vi "AR Drone Controller.vi"() -> ()   [LabVIEW 2014]
doc: "Very simple example showing how to use the base VIs to control the AR Drone and receive and display navigation data."
uses:
  <vilib>/LVH/AR Drone Toolkit/Decode NavData/Typedefs/NavData Demo.ctl
  Control 1.ctl
  <vilib>/LVH/AR Drone Toolkit/AR Drone.lvlib
panel:
  out "Video Stream":picture
  out "Battery Remaining":T1 scale=0.0..100.0
  out "NavData Out":T2
  in  "Control Cluster":T3 {"Yaw Speed" scale=-1.0..1.0; "Vertical Speed" scale=-1.0..1.0; "Pitch" scale=-1.0..1.0; "Roll" scale=-1.0..1.0}
  in  "stop":bool
  in  "Emergency Landing":bool
  in  "Take Off/Land":bool
  in  "Hover":bool
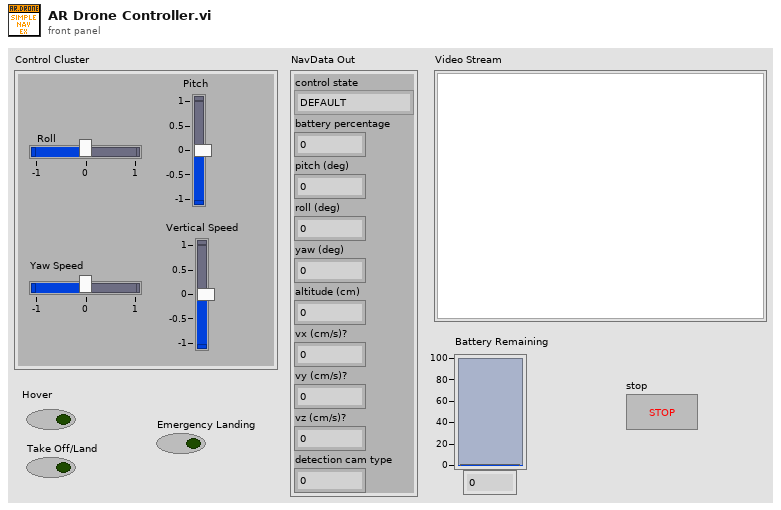
[diagram p1: front panel]
types:
  T1 = typedef "Control 1.ctl" = dbl
  T2 = typedef "AR Drone.lvlib/NavData Demo.ctl" = cluster{"control state":enum32{"DEFAULT", "INIT", "LANDING", "FLYING", "HOVERING", "TEST", "TRANS_TAKEOFF", "TRANS_GOTOFIX", "TRANS_LANDING"}, "battery percentage":u32, "pitch (deg)":sgl, "roll (deg)":sgl, "yaw (deg)":sgl, "altitude (cm)":u32, "vx (cm/s)?":sgl, "vy (cm/s)?":sgl, "vz (cm/s)?":sgl, "detection cam type":u32}
  T3 = cluster{"Roll":sgl, "Pitch":sgl, "Vertical Speed":sgl, "Yaw Speed":sgl}
  T4 = typedef "AR Drone.lvlib/AR Drone Resource.ctl" = cluster{"UDP Control Connection":refnum<k16>, "UDP NavData Connection":refnum<k16>, "UDP Video Connection (Drone 1.0)":refnum<k16>, "TCP Video Connection (Drone 2.0)":refnum<k5>, "TCP Control Port Connection":refnum<k5>, "Drone IP address":string, "Drone Command Port":u16, "Drone NavData Port":u16, "Drone Vid Stream Port":u16, "Drone TCP Control Port":u16, "Home IP address":string, "Home Command Port":u16, "Home NavData Port":u16, "Home Vid Stream Port":u16, "Drone Version":i32}
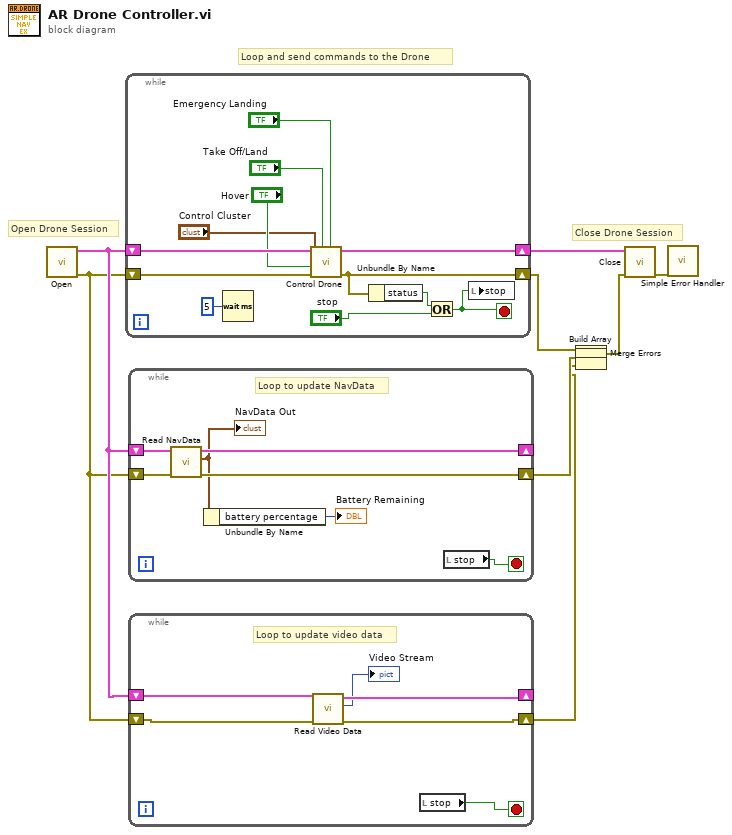
[diagram p0: block diagram]
diagram:
  # "Close Drone Session"
  # "Loop and send commands to the Drone"
  # "Open Drone Session"
  n1 = call <vilib>:"Open.vi"() -> ("error out"=w1:errorcluster, "AR Drone Resource"=w5:T4)  [unwired: 10 in]
  n2 = while {
    shift-right: [w16] -> w9
    shift-left: w5 -> [w20]
    shift-right: [w11] -> w8
    shift-left: w1 -> [w21]
    stop <- w10 stop-if-true
    n3 = Wait (ms)(milliseconds to wait=u32 5) -> ()  [unwired: 1 out]
    n4 = call <vilib>:"Control Drone.vi"("Emergency Landing"="Emergency Landing", "Takeoff/Land"="Take Off/Land", "error in (no error)"=w21, "Hover"="Hover", "Control Cluster"="Control Cluster", "AR Drone Resource"=w20) -> ("error out"=w11:errorcluster, "AR Drone Resource Out"=w16:T4)  [unwired: 4 in]
    n5 = Unbundle By Name(w11) -> ("status"=w13:bool)
    n6 = Or(x=w13, y="stop") -> (x .or. y?=w10:bool)
    n7 = local write "stop"(w10) -> ()
  }
  n8 = while {
    shift-right: [w26] -> _
    shift-left: w5 -> [w27]
    shift-right: [w24] -> w3
    shift-left: w1 -> [w25]
    stop <- w28 stop-if-true
    # "Loop to update NavData"
    n9 = call <vilib>:"Read NavData.vi"("error in (no error)"=w25, "AR Drone Resource"=w27) -> ("error out"=w24:errorcluster, "NavData Out"=w23:T2, "AR Drone Resource Out"=w26:T4)  [unwired: 7 in]
    "NavData Out" <- w23
    n10 = Unbundle By Name(w23) -> ("battery percentage"=→"Battery Remaining":u32)
    n11 = local read "stop"() -> (w28:bool)
  }
  n12 = while {
    shift-right: [w31] -> _
    shift-left: w5 -> [w33]
    shift-right: [w30] -> w2
    shift-left: w1 -> [w32]
    stop <- w34 stop-if-true
    # "Loop to update video data"
    n13 = call <vilib>:"Read Video Data.vi"("error in (no error)"=w32, "AR Drone Resource"=w33) -> ("error out"=w30:errorcluster, "Video Stream"=→"Video Stream":picture, "AR Drone Resource Out"=w31:T4)  [unwired: 7 in]
    n14 = local read "stop"() -> (w34:bool)
  }
  n15 = Build Array(w8, w3, w2) -> (w4:errorcluster[])
  n16 = Merge Errors(w4) -> (w7:errorcluster)
  n17 = call <vilib>:"Close.vi"("error in (no error)"=w7, "AR Drone Resource"=w9) -> ("error out"=w6:errorcluster)  [unwired: 9 in]
  n18 = call <vilib>:"Simple Error Handler.vi"("error in (no error)"=w6) -> ()  [unwired: 4 in, 5 out]
